vi "operational.vi"(2 "error out 4":errorcluster, 3 "VISA resource name 4":refnum<visa-resource-name>) -> (0 "error out 5":errorcluster, 1 "VISA resource name 5":refnum<visa-resource-name>)   [LabVIEW 2017]
panel:
  out "Boolean 3":bool
  out "String":string
  out "read buffer 3":string
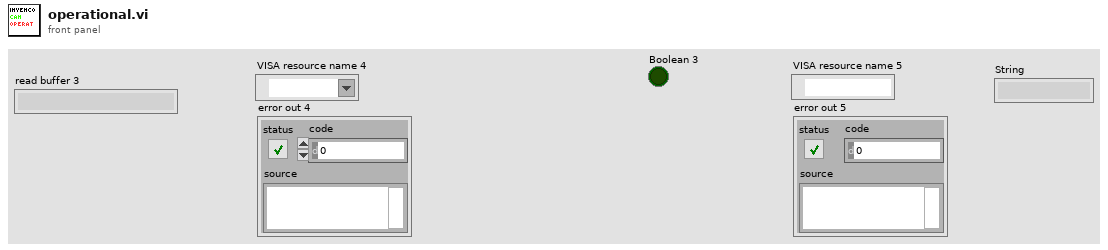
[diagram p1: front panel]
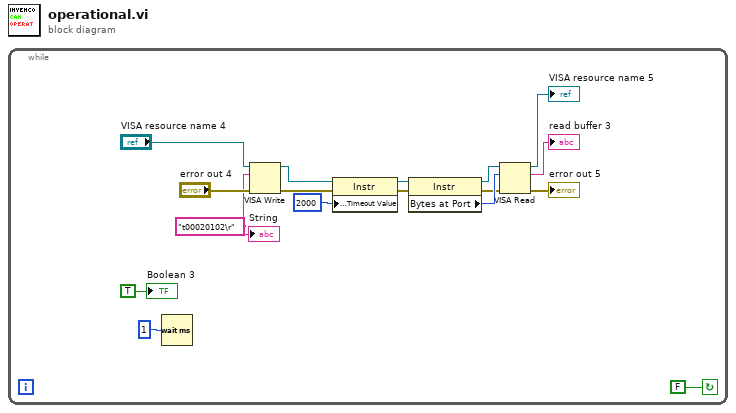
[diagram p0: block diagram]
diagram:
  n1 = while {
    stop <- FALSE continue-if-true
    w12 = "t00020102\r"
    n2 = Wait (ms)(milliseconds to wait=u32 1 ("millisecond multiple")) -> ()  [unwired: 1 out]
    n3 = VISA Write(VISA resource name="VISA resource name 4", write buffer=w12, error in (no error)="error out 4") -> (VISA resource name out=w7:refnum<visa-resource-name>, error out=w6:errorcluster)  [unwired: 1 out]
    n4 = property class="Instr"(reference=w7, error in=w6, "General Settings:Timeout Value"=u32 2000) -> (reference out=w4:refnum<visa-resource-name>, error out=w5:errorcluster)
    n5 = property class="Instr"(reference=w4, error in=w5) -> (reference out=w10:refnum<visa-resource-name>, error out=w9:errorcluster, "Bytes at Port"=w11:u32)
    n6 = VISA Read(VISA resource name=w10, byte count=w11, error in (no error)=w9) -> (VISA resource name out=→"VISA resource name 5":refnum<visa-resource-name>, read buffer=→"read buffer 3":string, error out=→"error out 5":errorcluster)  [unwired: 1 out]
    "String" <- w12
    "Boolean 3" <- TRUE
  }
